vi "显示测试结果-左上角-非存档数据输入.vi"(6 "单个数据结果":bool[](array[boolean])=[TRUE, TRUE, TRUE], 8 "显示坐标":cluster{dbl, "Numeric":dbl}[](array[cluster])=[{100.0, "Numeric"=300.0}, {100.0, "Numeric"=500.0}, {100.0, "Numeric"=700.0}, {100.0, "Numeric"=540.0}, {100.0, "Numeric"=620.0}, {100.0, "Numeric"=700.0}, {100.0, "Numeric"=780.0}, {100.0, "Numeric"=860.0}, {100.0, "Numeric"=940.0}], 9 "量测项目名称":string[](array[string]), 10 "显示数据":dbl[](array[numeric]), 11 "Img输入":T1) -> (3 "Image Out":T1)   [LabVIEW 2014]
uses:
  <vilib>/vision/Image Controls.llb/IMAQ Image.ctl
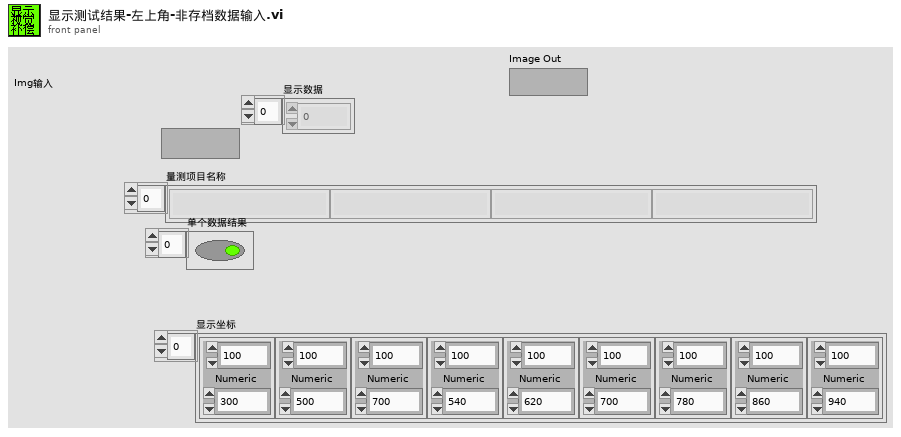
[diagram p1: front panel]
types:
  T1 = typedef "IMAQ Image.ctl" = refnum<image>
  T2 = cluster{"Desired Font (Application)":enum16{"User-specified Font", "Application Font", "System Font", "Dialog Font"}, "[User-specified Font]":cluster{"Font Name":string, "Size":i16, "Strikeout?":bool, "Italic?":bool, "Underline?":bool, "Outline?":bool, "Shadow?":bool, "Bold?":bool, "Rotation Angle":dbl}, "Horizontal Alignment":i16, "Vertical Alignment":i16}
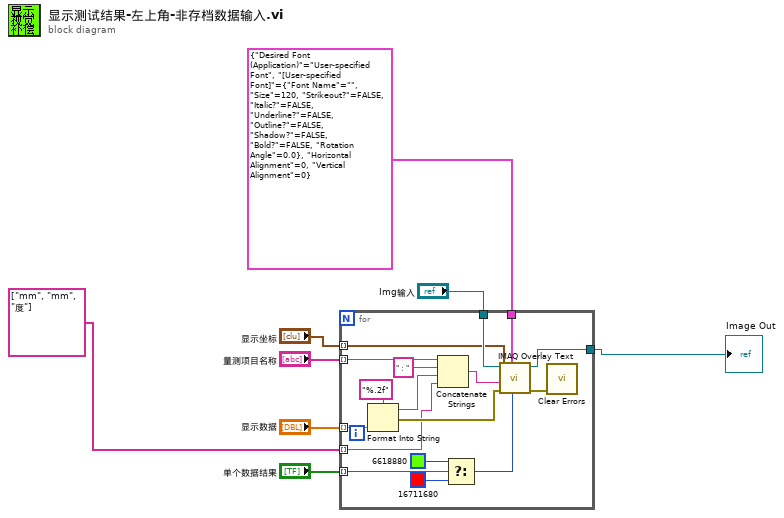
[diagram p0: block diagram]
diagram:
  n1 = for {
    tunnel: "Img输入" -> [w25]
    tunnel: "显示数据" -> [w24] mode=indexing
    tunnel: "显示坐标" -> [w23] mode=indexing
    tunnel: T2 {"Desired Font (Application)"=enum."User-specified Font", "[User-specified Font]"={"Font Name"="", "Size"=120, "Strikeout?"=FALSE, "Italic?"=FALSE, "Underline?"=FALSE, "Outline?"=FALSE, "Shadow?"=FALSE, "Bold?"=FALSE, "Rotation Angle"=0.0}, "Horizontal Alignment"=0, "Vertical Alignment"=0} ("Font, Size & Style") -> [w22]
    tunnel: "量测项目名称" -> [w18] mode=indexing
    tunnel: "单个数据结果" -> [w14] mode=indexing
    tunnel: [w10] -> w1
    tunnel: string[] ["mm", "mm", "度"] -> [w9] mode=indexing
    n2 = Format Into String(format string="%.2f" ("格式字符串"), w24) -> (resulting string=w16:string, error out=w20:errorcluster)  [unwired: 2 in]
    n3 = Concatenate Strings(w18, "：" ("字符串"), w16, w9) -> (w17:string)
    n4 = Select(t=u32 6618880 ("Text Color (black)"), s=w14, f=u32 16711680 ("Text Color (black)")) -> (s? t:f=w12:u32)
    n5 = call "IMAQ Overlay Text"("Text Color (black)"=w12, "Font, Size & Style"=w22, "error in (no error)"=w20, "String"=w17, "Origin"=w23, "Image"=w25) -> ("error out"=w19:errorcluster, "Image Out"=w10:T1)  [unwired: 4 in]
    n6 = call <vilib>:"Clear Errors.vi"("error in (no error)"=w19) -> ()  [unwired: 5 in, 2 out]
  }
  "Image Out" <- w1
